vi "com port send response test 1.vi"(0 "VISA Send port":refnum<visa-resource-name>, 1 "Wait for response msecs":u32=750, 2 "Comparison type":T1=enum."String in response somewhere", 5 "Send text":string, 7 "Expected response":string, 9 "Log in":string, 11 "error in (no error)":errorcluster, 12 "PassFail_In":bool=TRUE, 13 "Verbose on Errors?":bool=TRUE) -> (4 "VISA Send port out":refnum<visa-resource-name>, 6 "Response":string, 10 "Log out":string, 14 "PassFail_Out":bool, 15 "error out":errorcluster)   [LabVIEW 2013]
uses:
  Test Support VI/String compare type.ctl
panel:
  in  "Wait Msecs After cmd":u32=250
  out "Bytes at port":u32
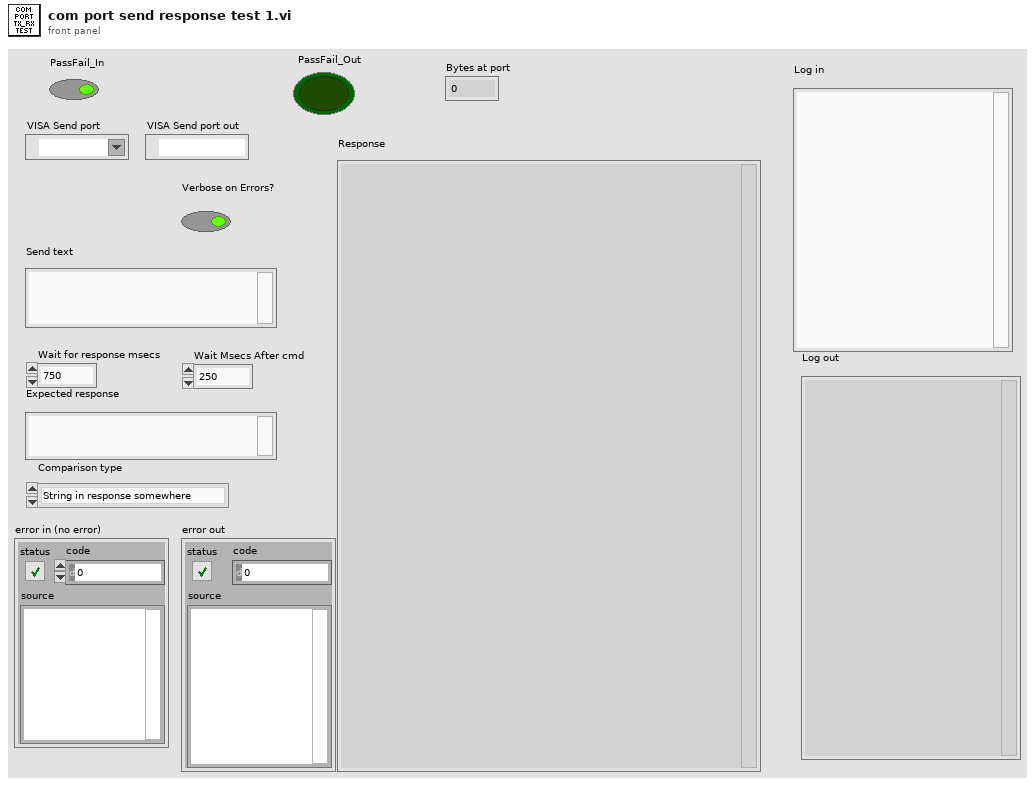
[diagram p1: front panel]
types:
  T1 = typedef "String compare type.ctl" = enum16{"String is exactly response", "String in response somewhere", "String not in response"}
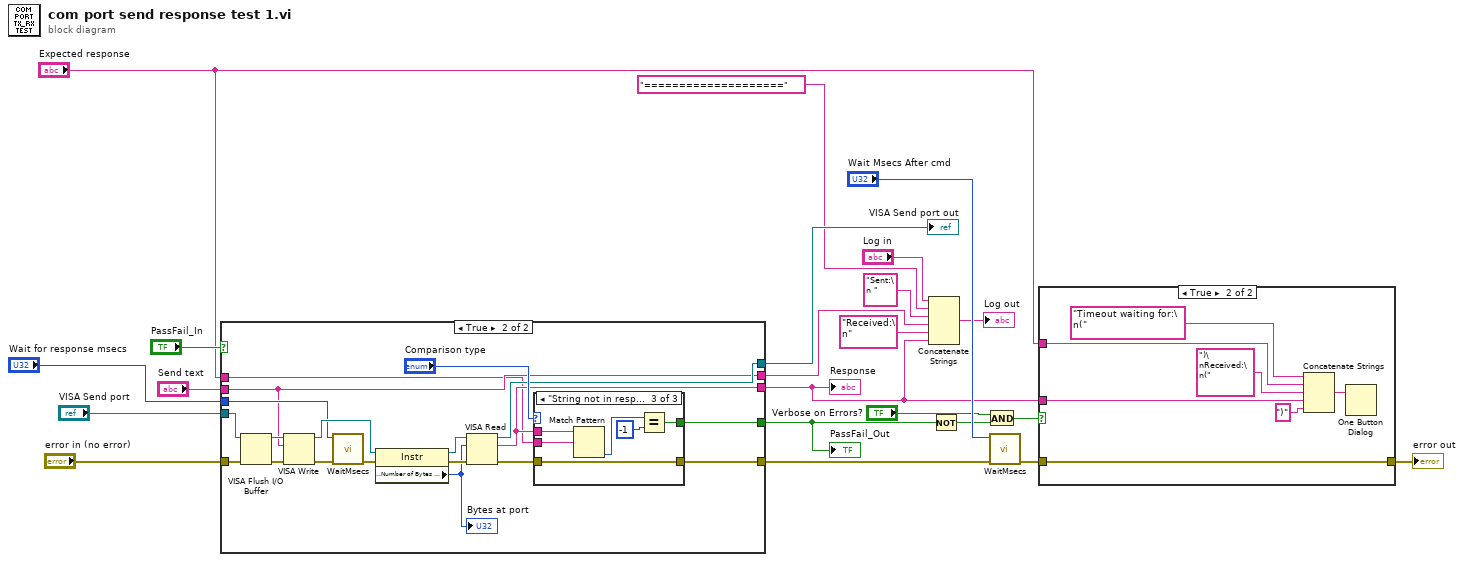
[diagram p0: block diagram]
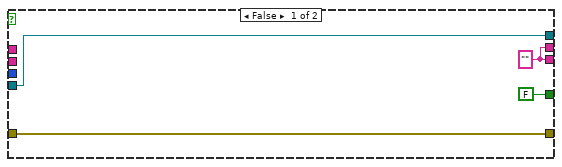
[diagram p3: hidden frame]
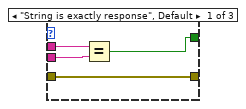
[diagram p4: hidden frame]
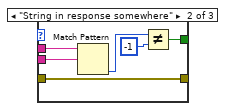
[diagram p5: hidden frame]
diagram:
  n1 = case shown="True" "PassFail_In" {
    tunnel: [FALSE w37] -> w6
    tunnel: "VISA Send port" -> [w24 w34]
    tunnel: [w25 w33] -> w17
    tunnel: "error in (no error)" -> [w25 w36]
    tunnel: [w24 w31] -> w19
    tunnel: "Wait for response msecs" -> [_ w30]
    tunnel: "Send text" -> [_ w28]
    tunnel: [w23 w29] -> w3
    tunnel: [w23 w28] -> w12
    tunnel: "Expected response" -> [_ w27]
    frame False {
      w23 = "" ("read buffer")
    }
    frame True {
      n2 = VISA Flush I/O Buffer(VISA resource name=w34, error in (no error)=w36) -> (VISA resource name out=w44:refnum<visa-resource-name>, error out=w45:errorcluster)  [unwired: 1 in]
      n3 = VISA Write(VISA resource name=w44, write buffer=w28, error in (no error)=w45) -> (VISA resource name out=w32:refnum<visa-resource-name>, error out=w43:errorcluster)  [unwired: 1 out]
      n4 = call "WaitMsecs.vi"("error in (no error)"=w43, "Wait Msecs"=w30) -> ("error out"=w42:errorcluster)  [unwired: 9 in]
      n5 = property class="Instr"(reference=w32, error in=w42) -> (reference out=w39:refnum<visa-resource-name>, error out=w41:errorcluster, "Serial Settings:Number of Bytes at Serial Port"=w40:u32)
      "Bytes at port" <- w40
      n6 = VISA Read(VISA resource name=w39, byte count=w40, error in (no error)=w41) -> (VISA resource name out=w31:refnum<visa-resource-name>, read buffer=w29:string, error out=w35:errorcluster)  [unwired: 1 out]
      n7 = case shown="\"String not in response\"" "Comparison type" {
        tunnel: w29 -> [w49 w55 w59]
        tunnel: w35 -> [w46 w50 w56]
        tunnel: w27 -> [w48 w54 w58]
        tunnel: [w47 w51 w57] -> w37
        tunnel: [w46 w50 w56] -> w33
        frame "String is exactly response", Default {
          n8 = Equal?(x=w49, y=w48) -> (x = y?=w47:bool)
        }
        frame "String in response somewhere" {
          n9 = Match Pattern(string=w55, regular expression=w54) -> (offset past match=w53:i32)  [unwired: 1 in, 3 out]
          n10 = Not Equal?(x=w53, y=-1) -> (x != y?=w51:bool)
        }
        frame "String not in response" {
          n11 = Match Pattern(string=w59, regular expression=w58) -> (offset past match=w61:i32)  [unwired: 1 in, 3 out]
          n12 = Equal?(x=w61, y=-1) -> (x = y?=w57:bool)
        }
      }
    }
  }
  "PassFail_Out" <- w6
  "VISA Send port out" <- w19
  "Response" <- w3
  n13 = Concatenate Strings("Log in", "====================" ("string"), "Sent:\n " ("string"), w12, "Received:\n" ("string"), w3) -> (→"Log out":string)
  n14 = Not(x=w6) -> (.not. x?=w7:bool)
  n15 = And(x="Verbose on Errors?", y=w7) -> (x .and. y?=w5:bool)
  n16 = call "WaitMsecs.vi"("error in (no error)"=w17, "Wait Msecs"="Wait Msecs After cmd") -> ("error out"=w1:errorcluster)  [unwired: 9 in]
  n17 = case shown="True" w5 {
    tunnel: "Expected response" -> [_ w68]
    tunnel: w3 -> [_ w66]
    tunnel: [w62 w63] -> w2
    tunnel: w1 -> [w62 w63]
    frame False {
    }
    frame True {
      n18 = Concatenate Strings("Timeout waiting for:\n(" ("string"), w68, ")\nReceived:\n(" ("string"), w66, ")" ("string")) -> (w64:string)
      n19 = One Button Dialog(message=w64) -> ()  [unwired: 1 in, 1 out]
    }
  }
  "error out" <- w2
